vi "Advanced HTML Documentation Wizard.vi"(11 "error in (no error)":errorcluster) -> (15 "error out":errorcluster)   [LabVIEW 2012]
doc: "VI Description text"
uses:
  _Controls and TypeDefs/StartPathLocation_enum.ctl
  _Controls and TypeDefs/InfoFromOldHTML_cluster.ctl
  _Controls and TypeDefs/UserDialogStates.ctl
  <vilib>/Platform/browser.llb/Open URL in Default Browser (string).vi
  <vilib>/Platform/browser.llb/Open URL in Default Browser (path).vi
panel:
  in  "www.labicom.net":bool
  in  "IsChildrenTable?":bool
  in  "Table":string[][](table)=[[" "]] caption="Table with a list of children VIs (that current VI contains)"
  in  "IsScrollableDetails?":bool=TRUE
  in  "Help Button":bool
  out "LV <help> directory?":bool
  in  "IsDetailedHelpLink?":bool=TRUE
  in  "Info extracted from old HTML":T1={"_vi_name_"="", "_vi_description_text_"="", "_vi_controls_and_indicators_descriptions_"="", "_name_of_owning_library_"="", "_owning_library_html_"="", "_Packages_"="Base Package", "_Platforms_"="Windows", "_details_text_"="Put details here", "_example_screenshot_"="", "_example_vi_"="", "_path_to_example_file_"=path "", "IsDetailsON?"=FALSE, "IsOwningLibraryON?"=FALSE, "IsExamplesON?"=FALSE, "IsTableON?"=FALSE, "IsScrollableON?"=FALSE, "IsDetailedHelpLinkON?"=FALSE, "Table Objects array"=[], "Table Descriptions array"=[], "Table Links array"=[], "Start path location"=enum."VI folder"}
  in  "Next_btn":bool caption="Produce VI documentation"
  out "HTML File Path":path
  in  "Cancel Button":bool
  out "Cancelled by User?":bool
  in  "Examples_chkBox":bool
  in  "Details_chkBox":bool=TRUE
  in  "OwningLibrary_chkBox":bool caption="Owning Library/Palette Information"
  in  "Name of Owning Library":string="Put a name here" caption="Name of Owning Library or Palette"
  in  "Path to Owning Library":string caption="Path to Owning Library or Palette"
  in  "Names of Packages":string="Base Package" caption="Names of libraries/packages that this VI requires for its operation"
  in  "Names of Platforms":string="Windows" caption="Names of platforms that this VI supports"
  in  "Details":string="Put details here"
  in  "Image Path for Example":string caption="Path to the image file for Example category"
  in  "Example VI name":string
  in  "Example VI Path":path
  in  "VI Description":string caption="VI Description (with HTML tags)"
  in  "Start path location":T2
  in  "Documentable VI Path":path
  # "Configure VI Documentation Layout"
  # "Additional layout elements for LabVIEW help"
  # "Caution: place <_caution_> into your text"
  # "Note: place <_note_> into your text"
  # "Tip: place <_tip_> into your text"
  # "Windows"
  # "Platform: enclose platform name between\n<_platform_> and </_platform_> tags"
  # "bold"
  # "Text in bold: enclose such text between\n<B> and </B> tags"
  # "Attention!"
  # "Caution Text: enclose such text between \n<_caution_text_> and </_caution_text_> tags"
  # "vigods.com"
  # "Link: place relative path in place of '_path_' and\ntext in place of '_text_' and insert resulting string\nwherever you need: \n<a href=\"_path_\">_text_</a>"
  # "monospace"
  # "Monospace: enclose such text between\n<_monospace_> and </_monospace_> tags"
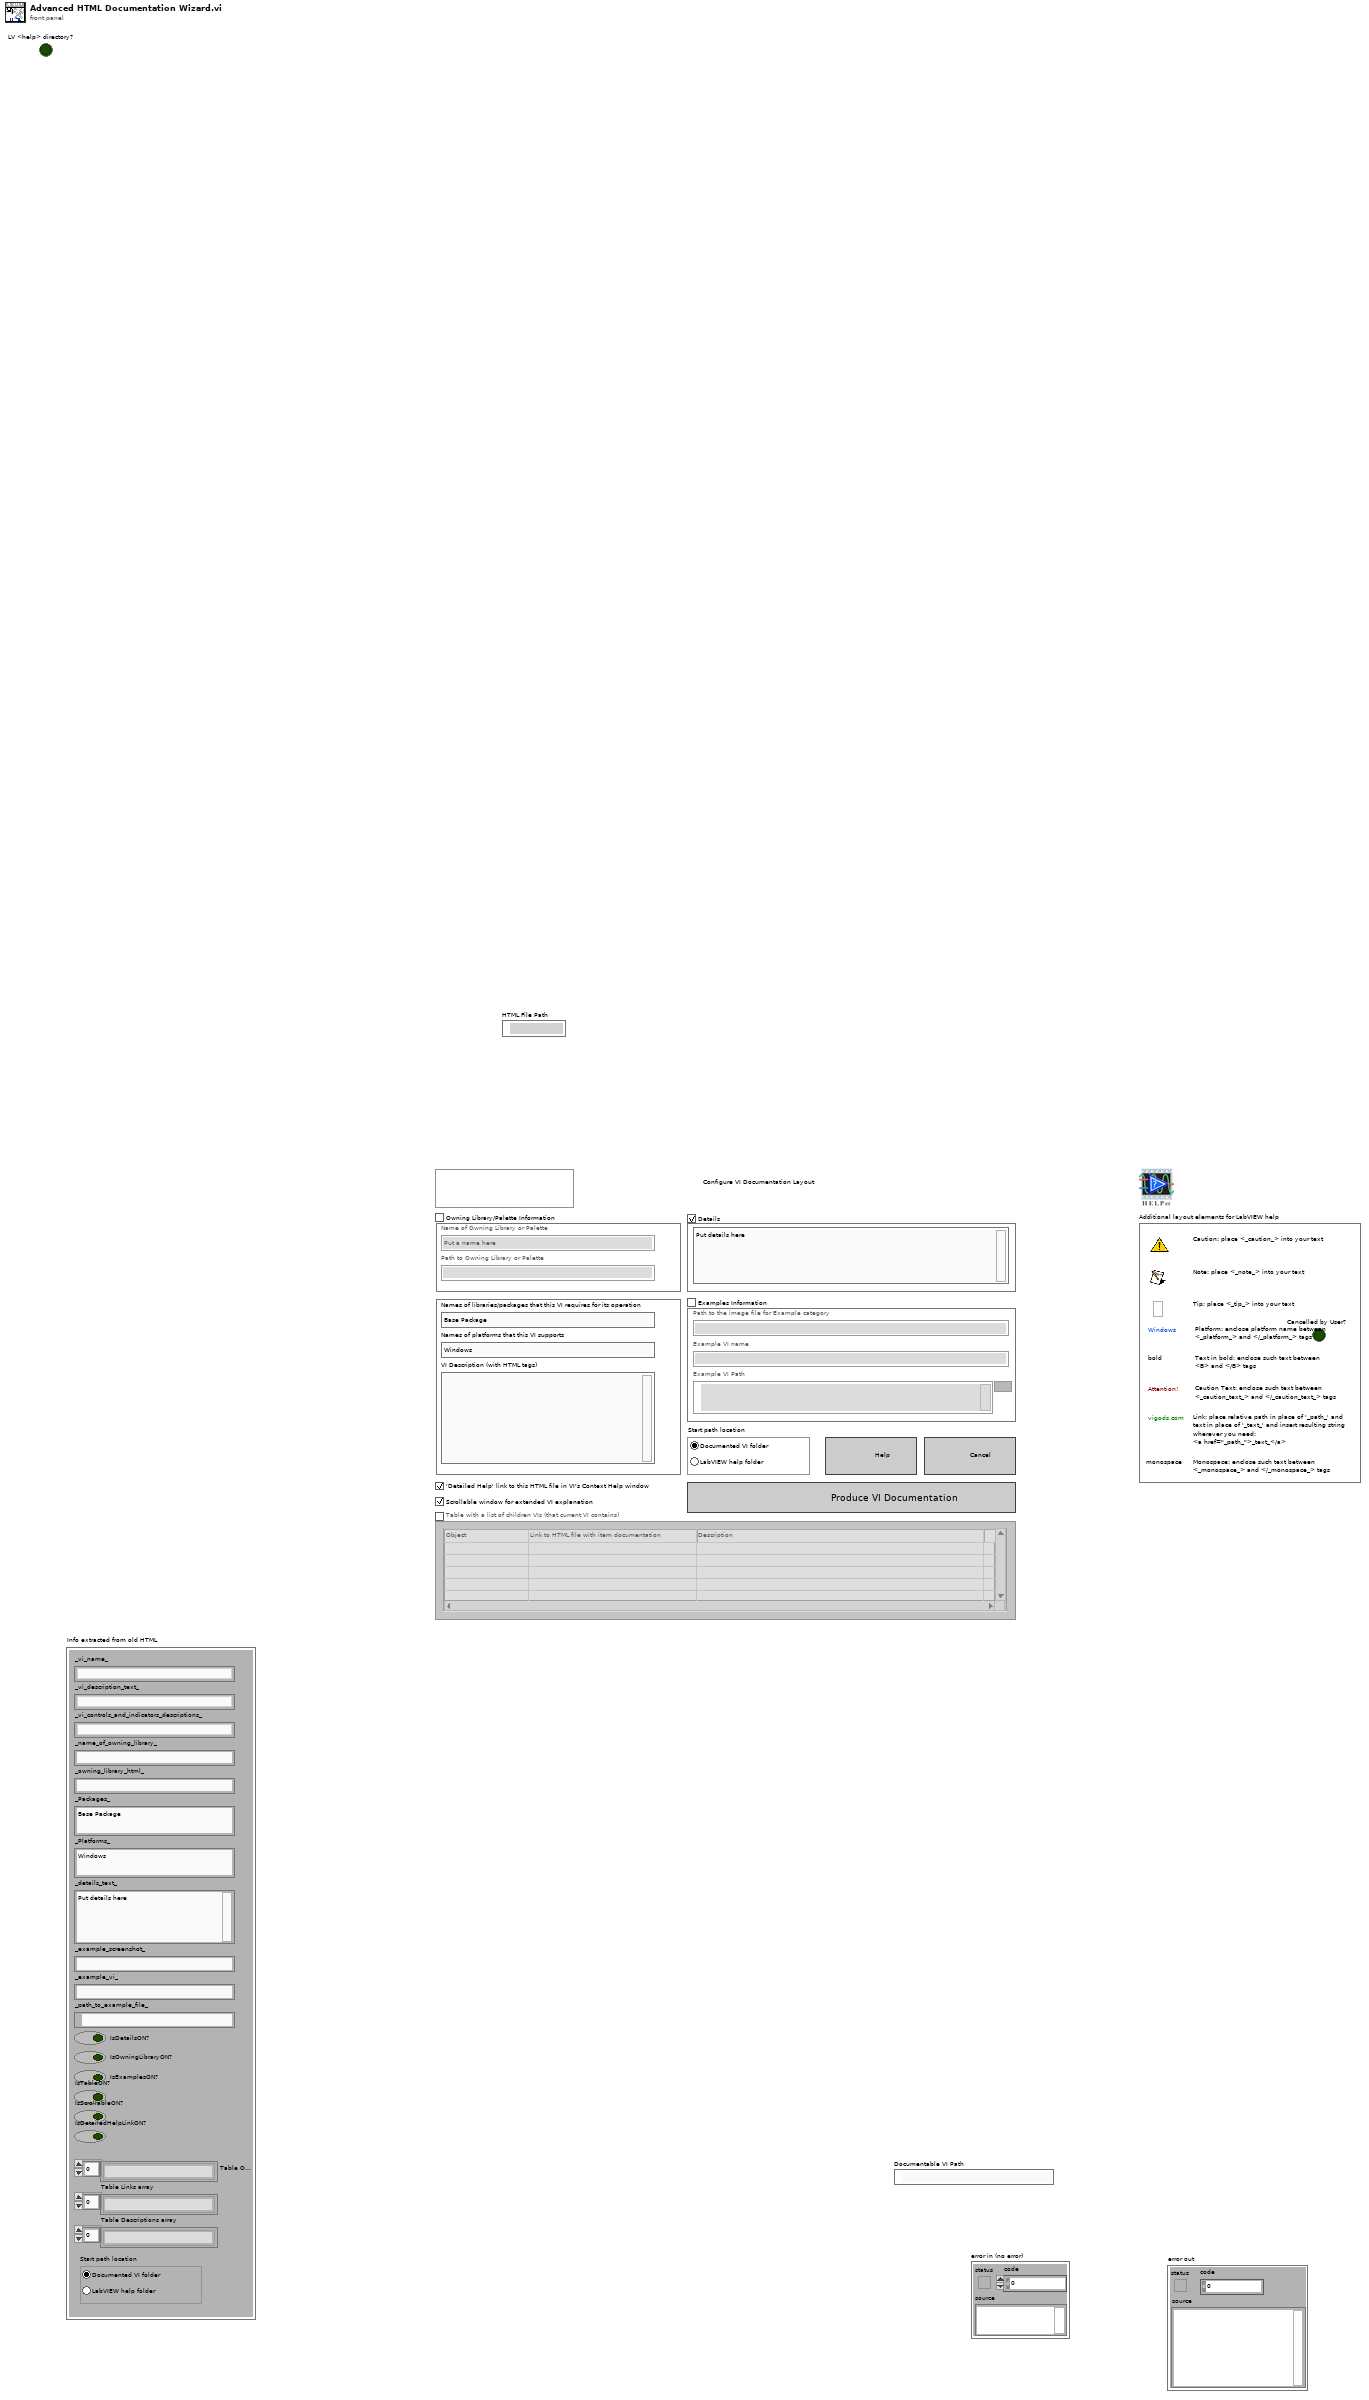
[diagram p1: front panel]
types:
  T1 = typedef "InfoFromOldHTML_cluster.ctl" = cluster{"_vi_name_":string, "_vi_description_text_":string, "_vi_controls_and_indicators_descriptions_":string, "_name_of_owning_library_":string, "_owning_library_html_":string, "_Packages_":string, "_Platforms_":string, "_details_text_":string, "_example_screenshot_":string, "_example_vi_":string, "_path_to_example_file_":path, "IsDetailsON?":bool, "IsOwningLibraryON?":bool, "IsExamplesON?":bool, "IsTableON?":bool, "IsScrollableON?":bool, "IsDetailedHelpLinkON?":bool, "Table Objects array":string[], "Table Descriptions array":string[], "Table Links array":string[], "Start path location":T2}
  T2 = typedef "StartPathLocation_enum.ctl" = enum32{"VI folder", "Help folder"}
  T3 = typedef "UserDialogStates.ctl" = enum16{"Overview", "Known Issues", "Choose parameters", "Update", "Choose HTML file path", "Choose Images directory path", "Decide if there is Context Help", "Choose help hierarchy", "Generate HTML", "Installation", "System Requirements", "Software Support", "Device Support", "Upgrade Issues", "New Features", "Fixed Issues", "Developer", "Contact Support", "Copyright", "Trademarks", "Patents", "Disclaimer", "Save", "Shutdown"}
  T4 = enum8{"Enabled", "Disabled", "Disabled and Grayed Out"}
  T5 = typedef "LVRowAndColumnTypeDef.ctl" = cluster{"Row":i32, "Column":i32}
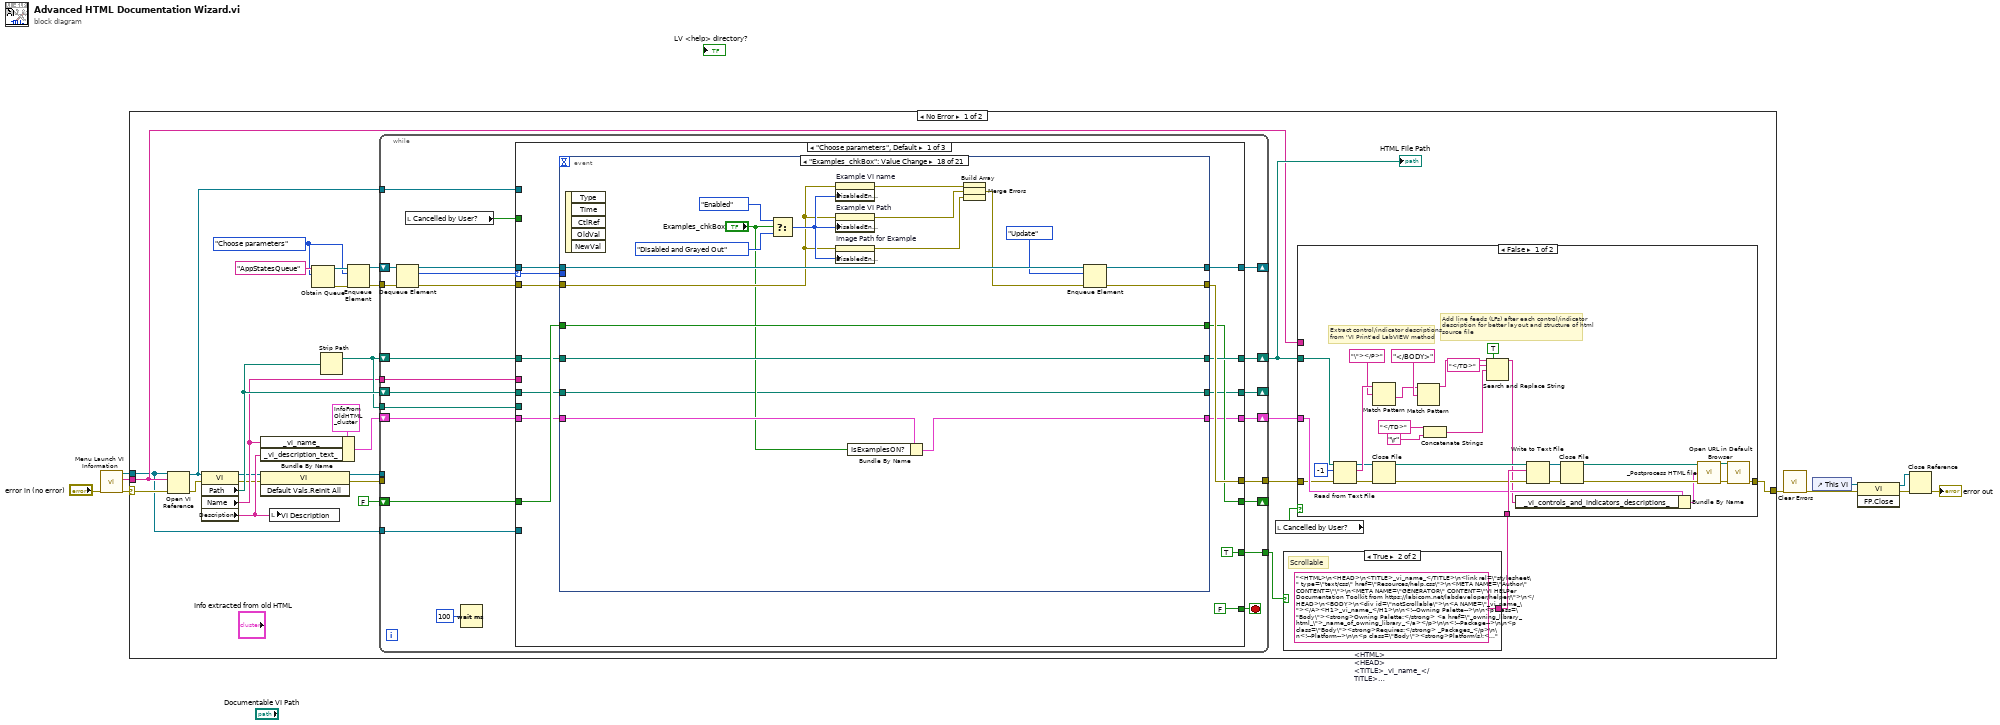
[diagram p0: block diagram]
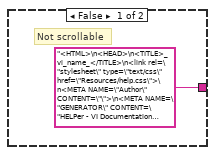
[diagram p2: hidden frame]
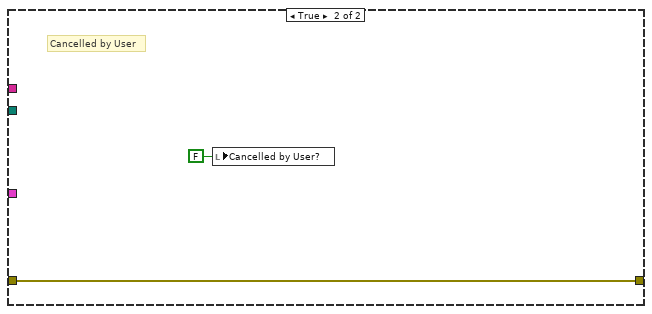
[diagram p3: hidden frame]
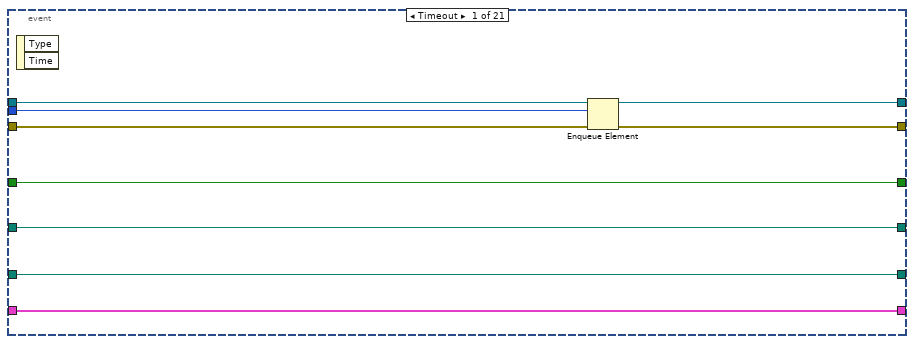
[diagram p4: hidden frame]
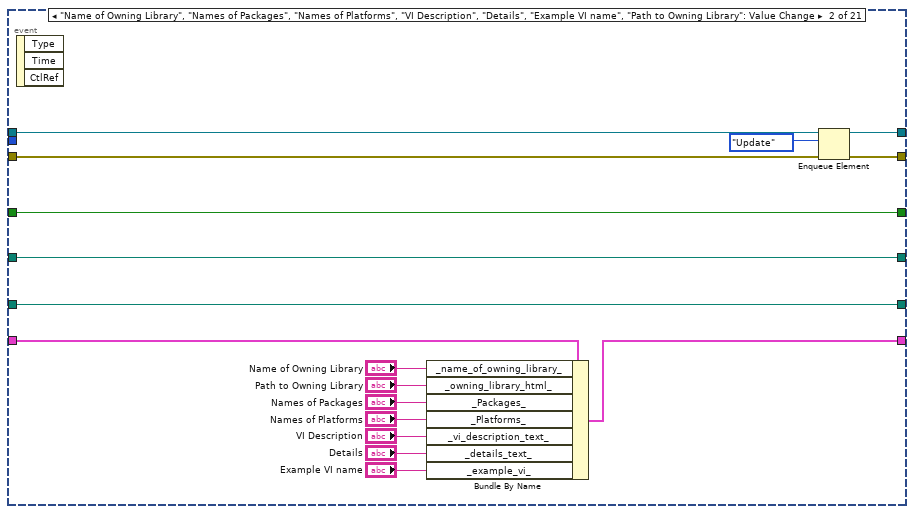
[diagram p5: hidden frame]
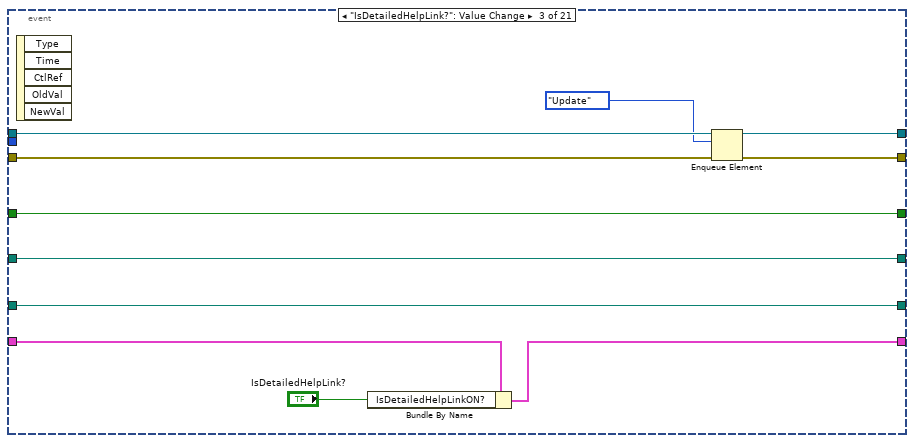
[diagram p6: hidden frame]
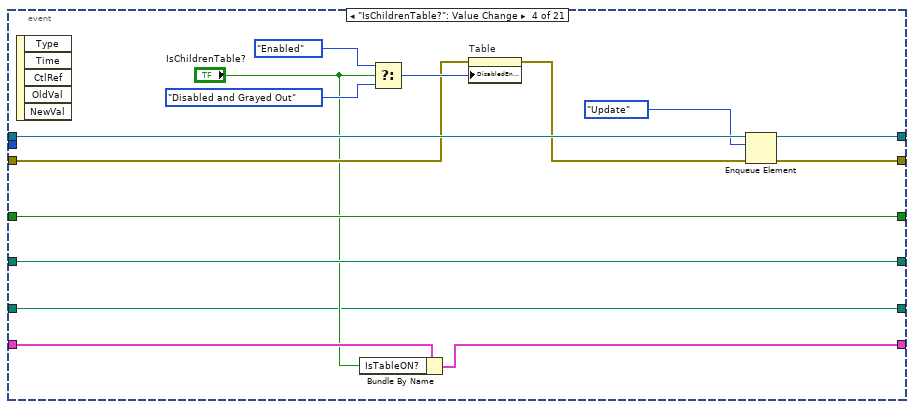
[diagram p7: hidden frame]
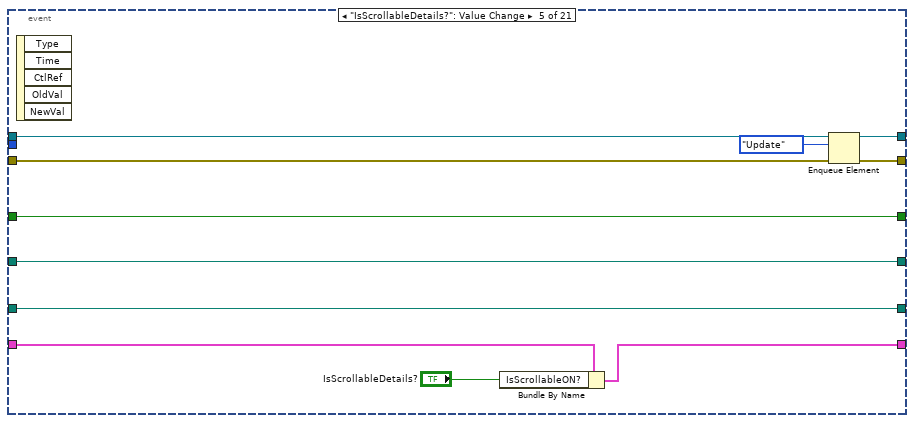
[diagram p8: hidden frame]
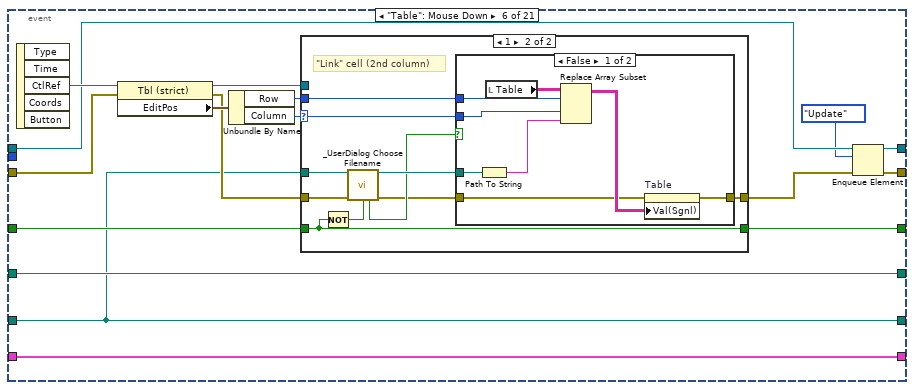
[diagram p9: hidden frame]
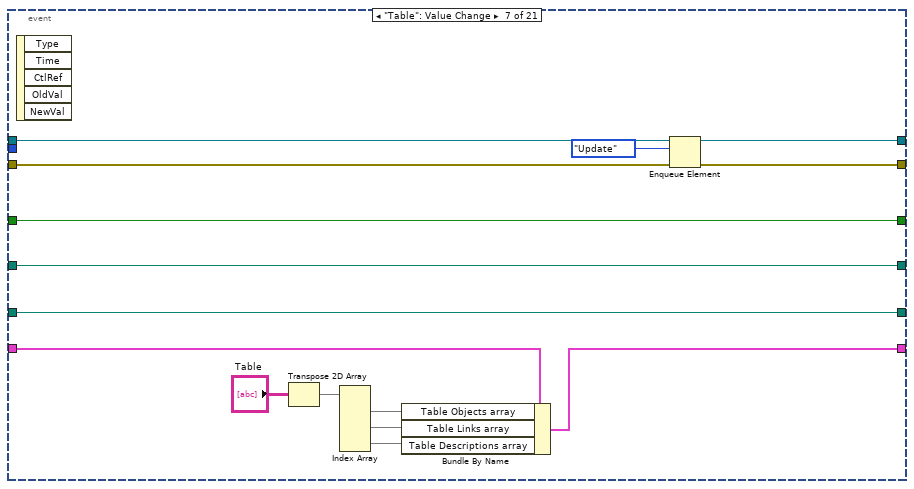
[diagram p12: hidden frame]
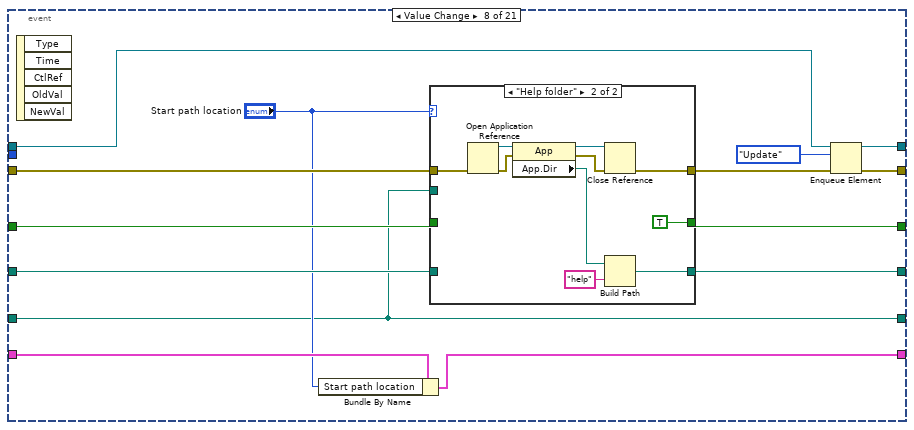
[diagram p13: hidden frame]
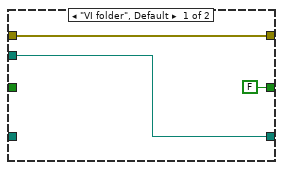
[diagram p14: hidden frame]
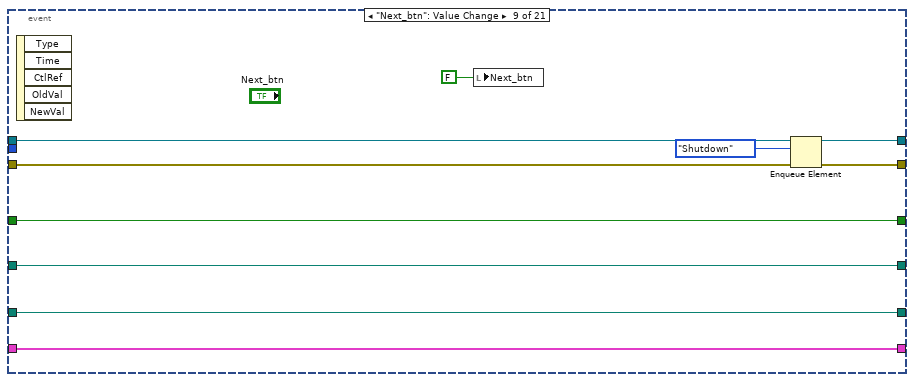
[diagram p15: hidden frame]
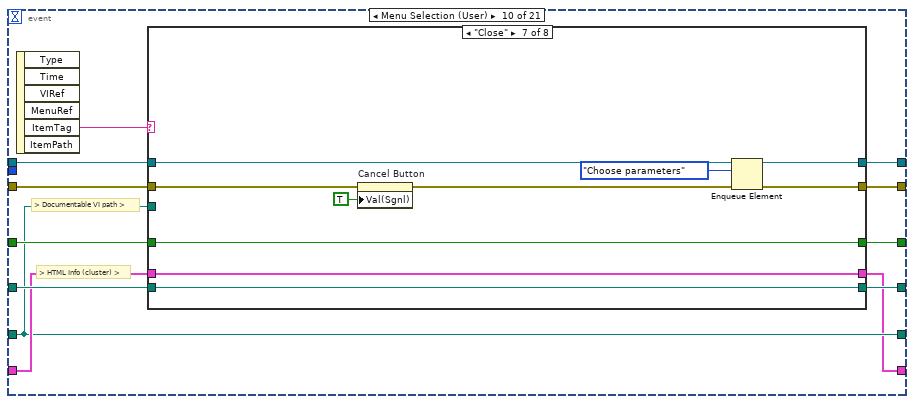
[diagram p16: hidden frame]
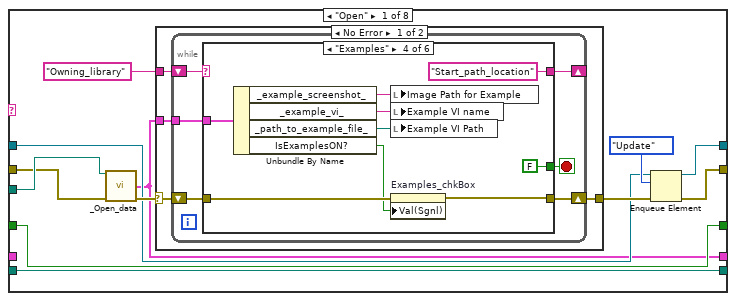
[diagram p17: hidden frame]
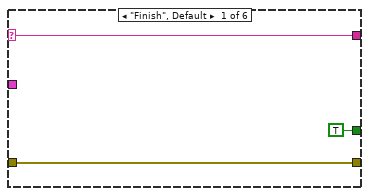
[diagram p18: hidden frame]
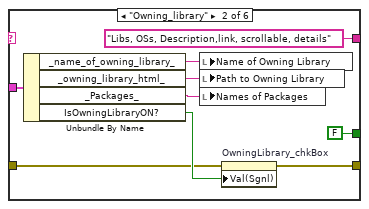
[diagram p19: hidden frame]
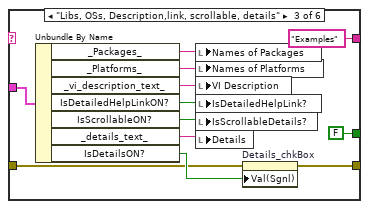
[diagram p20: hidden frame]
diagram:
  n1 = call <vilib>:"Menu Launch VI Information.vi"("error in (no error)"="error in (no error)") -> ("error out"=w7:errorcluster, "Menu Launch:VI"=w9:string, "Menu Launch:App"=w10:refnum<vi>)  [unwired: 8 in]
  n2 = case shown="No Error" w7 {
    selector: w7 -> [w37 w766]
    tunnel: w10 -> [w23 w765]
    tunnel: w9 -> [w24 _]
    tunnel: [w34 w764] -> w2
    frame No Error {
      w13 = UserDialogStates."Choose parameters" ("UserDialogSteps")
      n3 = Open VI Reference(application reference (local)=w23, vi path=w24, error in (no error)=w37) -> (vi reference=w25:refnum<vi>, error out=w39:errorcluster)  [unwired: 3 in]
      n4 = property class="VI"(reference=w25, error in=w39) -> (reference out=w22:refnum<vi>, error out=w20:errorcluster, "Path"=w28:path, "Name"=w26:string, "Description"=w30:string)
      n5 = Bundle By Name(cluster=T1 {"_vi_name_"="", "_vi_description_text_"="", "_vi_controls_and_indicators_descriptions_"="", "_name_of_owning_library_"="", "_owning_library_html_"="", "_Packages_"="Base Package", "_Platforms_"="Windows", "_details_text_"="Put details here", "_example_screenshot_"="", "_example_vi_"="", "_path_to_example_file_"=path "", "IsDetailsON?"=FALSE, "IsOwningLibraryON?"=FALSE, "IsExamplesON?"=FALSE, "IsTableON?"=FALSE, "IsScrollableON?"=FALSE, "IsDetailedHelpLinkON?"=FALSE, "Table Objects array"=[], "Table Descriptions array"=[], "Table Links array"=[], "Start path location"=enum."VI folder"} ("Info extracted from old HTML"), "_vi_name_"=w26, "_vi_description_text_"=w30) -> (w29:T1)
      n6 = invoke class="VI" method="Default Vals.Reinit All"(reference=w22, error in=w20) -> (reference out=w19:refnum<vi>, error out=w21:errorcluster)  [unwired: 1 in, 1 out]
      n7 = local write "VI Description"(w30) -> ()
      n8 = Obtain Queue(name (unnamed)="AppStatesQueue", element data type=w13) -> (queue out=w14:refnum<queue>, error out=w15:errorcluster)  [unwired: 3 in, 1 out]
      n9 = Strip Path(path=w28) -> (stripped path=w27:path)  [unwired: 1 out]
      n10 = Enqueue Element(queue=w14, element=w13, error in (no error)=w15) -> (queue out=w12:refnum<queue>, error out=w11:errorcluster)  [unwired: 1 in, 1 out]
      n11 = while {
        shift-right: [w92] -> _
        shift-left: w12 -> [w75]
        tunnel: w27 -> [w91]
        shift-right: [w90] -> w32
        shift-left: w27 -> [w89]
        shift-right: [w87] -> w35
        shift-left: w29 -> [w88]
        tunnel: w21 -> [_]
        shift-right: [w83] -> _
        shift-left: FALSE -> [w86]
        shift-right: [w82] -> _
        shift-left: w28 -> [w85]
        tunnel: [w84] -> w33
        tunnel: w26 -> [w80]
        tunnel: w25 -> [w79]
        tunnel: w23 -> [w78]
        tunnel: w19 -> [_]
        tunnel: [w77] -> w17
        tunnel: w11 -> [w76]
        stop <- w94 stop-if-true
        n12 = Dequeue Element(queue=w75, error in (no error)=w76) -> (queue out=w72:refnum<queue>, element=w74:T3, error out=w73:errorcluster)  [unwired: 1 in, 1 out]
        n13 = local read "Cancelled by User?"() -> (w81:bool)
        n14 = Wait (ms)(milliseconds to wait=u32 100) -> ()  [unwired: 1 out]
        n15 = case shown="\"Choose parameters\", Default" w74 {
          selector: w74 -> [w108 _ w621]
          tunnel: [FALSE FALSE w633] -> w94
          tunnel: [w107 w611 w627] -> w92
          tunnel: w91 -> [_ _ _]
          tunnel: [w103 w609 w625] -> w90
          tunnel: w89 -> [w104 w609 w628]
          tunnel: w88 -> [w100 w607 w631]
          tunnel: [w95 w607 w630] -> w87
          tunnel: w86 -> [w105 w606 w624]
          tunnel: w85 -> [w97 w608 w632]
          tunnel: [w106 w610 w629] -> w84
          tunnel: [w102 w606 w623] -> w83
          tunnel: [w96 w608 w626] -> w82
          tunnel: w81 -> [_ _ w622]
          tunnel: w80 -> [_ _ w618]
          tunnel: w79 -> [_ _ w620]
          tunnel: w78 -> [_ _ w619]
          tunnel: [TRUE ("IsScrollableDetails?") TRUE ("IsScrollableDetails?") w617] -> w77
          tunnel: w73 -> [w99 w614 w616]
          tunnel: w72 -> [w98 w613 w615]
          frame "Choose parameters", Default {
            n16 = event shown="[17] \"Examples_chkBox\": Value Change" {
              selector: _ -> [_ _ _ _ _ _ _ _ _ _ _ _ _ _ _ _ _ _ _ _ _]
              dyn-events: _ -> [_ _ _ _ _ _ _ _ _ _ _ _ _ _ _ _ _ _ _ _ _]
              timeout: _ -> [_ _ _ _ _ _ _ _ _ _ _ _ _ _ _ _ _ _ _ _ _]
              tunnel: w108 -> [w116 _ _ _ _ _ _ _ _ _ _ _ _ _ _ _ _ _ _ _ _]
              tunnel: [w114 w129 w141 w152 w165 w176 w220 w231 w256 w265 w434 w459 w476 w486 w513 w524 w541 w557 w573 w584 w596] -> w107
              tunnel: w105 -> [w117 w134 w145 w158 w170 w183 w224 w236 w260 w273 w438 w462 w474 w491 w509 w529 w546 w564 w580 w590 w601]
              tunnel: w99 -> [w113 w132 w143 w153 w167 w180 w222 w237 w259 w267 w442 w456 w477 w493 w512 w528 w544 w559 w578 w591 w598]
              tunnel: [w112 w130 w140 w151 w164 w175 w219 w230 w257 w269 w433 w458 w475 w485 w511 w523 w540 w556 w572 w583 w595] -> w106
              tunnel: w104 -> [w118 w135 w146 w157 w169 w181 w225 w239 w261 w271 w441 w465 w473 w492 w510 w532 w547 w565 w579 w589 w602]
              tunnel: [w118 w135 w146 w157 w169 w181 w225 w238 w261 w270 w441 w465 w473 w492 w510 w532 w547 w565 w579 w589 w602] -> w103
              tunnel: [w117 w134 w145 w158 w170 w182 w224 w235 w260 w272 w438 w462 w474 w491 w509 w529 w546 w564 w580 w590 w601] -> w102
              tunnel: w100 -> [w110 w128 w139 w150 w172 w173 w212 w229 w253 w268 w431 w453 w482 w483 w517 w522 w539 w555 w570 w581 w592]
              tunnel: w98 -> [w115 w133 w144 w156 w166 w178 w223 w233 w258 w266 w437 w460 w478 w490 w514 w527 w545 w561 w575 w586 w597]
              tunnel: w97 -> [w111 w127 w137 w148 w163 w174 w213 w227 w254 w264 w432 w454 w472 w484 w508 w520 w537 w553 w571 w582 w593]
              tunnel: [w111 w127 w137 w148 w163 w174 w213 w227 w254 w264 w432 w454 w472 w484 w508 w520 w537 w553 w571 w582 w593] -> w96
              tunnel: [w110 w126 w136 w147 w162 w173 w211 w226 w253 w263 w431 w453 w480 w483 w507 w519 w536 w552 w570 w581 w592] -> w95
              event Timeout {
                n17 = event-data() -> ()  [unwired: 1 in, 2 out]
                n18 = Enqueue Element(queue=w115, element=w116, error in (no error)=w113) -> (queue out=w114:refnum<queue>, error out=w112:errorcluster)  [unwired: 1 in, 1 out]
              }
              event "Name of Owning Library", "Names of Packages", "Names of Platforms", "VI Description", "Details", "Example VI name", "Path to Owning Library": Value Change {
                n19 = event-data() -> ()  [unwired: 1 in, 3 out]
                n20 = Bundle By Name(cluster=w128, "_name_of_owning_library_"="Name of Owning Library", "_owning_library_html_"="Path to Owning Library", "_Packages_"="Names of Packages", "_Platforms_"="Names of Platforms", "_vi_description_text_"="VI Description", "_details_text_"="Details", "_example_vi_"="Example VI name") -> (w126:T1)
                n21 = Enqueue Element(queue=w133, element=UserDialogStates."Update" ("UserDialogSteps"), error in (no error)=w132) -> (queue out=w129:refnum<queue>, error out=w130:errorcluster)  [unwired: 1 in, 1 out]
              }
              event "IsDetailedHelpLink?": Value Change {
                n22 = event-data() -> ()  [unwired: 1 in, 5 out]
                n23 = Bundle By Name(cluster=w139, "IsDetailedHelpLinkON?"="IsDetailedHelpLink?") -> (w136:T1)
                n24 = Enqueue Element(queue=w144, element=UserDialogStates."Update" ("UserDialogSteps"), error in (no error)=w143) -> (queue out=w141:refnum<queue>, error out=w140:errorcluster)  [unwired: 1 in, 1 out]
              }
              event "IsChildrenTable?": Value Change {
                n25 = event-data() -> ()  [unwired: 1 in, 5 out]
                n26 = Bundle By Name(cluster=w150, "IsTableON?"="IsChildrenTable?") -> (w147:T1)
                n27 = Select(t=T4."Enabled" ("Disabled"), s="IsChildrenTable?", f=T4."Disabled and Grayed Out") -> (s? t:f=w159:T4)
                n28 = property on="Table" class="Tbl (strict)"(error in=w153, "DisabledEnum"=w159) -> (error out=w154:errorcluster)  [unwired: 1 in, 1 out]
                n29 = Enqueue Element(queue=w156, element=UserDialogStates."Update" ("UserDialogSteps"), error in (no error)=w154) -> (queue out=w152:refnum<queue>, error out=w151:errorcluster)  [unwired: 1 in, 1 out]
              }
              event "IsScrollableDetails?": Value Change {
                n30 = event-data() -> ()  [unwired: 1 in, 5 out]
                n31 = Bundle By Name(cluster=w172, "IsScrollableON?"="IsScrollableDetails?") -> (w162:T1)
                n32 = Enqueue Element(queue=w166, element=UserDialogStates."Update" ("UserDialogSteps"), error in (no error)=w167) -> (queue out=w165:refnum<queue>, error out=w164:errorcluster)  [unwired: 1 in, 1 out]
              }
              event "Table": Mouse Down {
                n33 = event-data() -> ("CtlRef"=w184:refnum<vi>)  [unwired: 1 in, 4 out]
                n34 = property class="Tbl (strict)"(reference=w184, error in=w180) -> (reference out=w187:refnum<vi>, error out=w186:errorcluster, "EditPos"=w189:T5)
                n35 = Unbundle By Name(w189) -> ("Row"=w185:i32, "Column"=w188:i32)
                n36 = case shown="1" w188 {
                  selector: w188 -> [_ w197]
                  tunnel: w183 -> [w190 w196]
                  tunnel: w174 -> [_ w201]
                  tunnel: w187 -> [_ _]
                  tunnel: w186 -> [w191 w199]
                  tunnel: w185 -> [_ w198]
                  tunnel: [w191 w192] -> w179
                  tunnel: [w190 w196] -> w182
                  frame 0, Default {
                  }
                  frame 1 {
                    # "\"Link\" cell (2nd column)"
                    n37 = Not(x=w196) -> (.not. x?=w195:bool)
                    n38 = call "_UserDialog Choose Filename.vi"("VI Default Path"=w201, "error in (no error)"=w199, "Not In <help> directory? (Yes: T)"=w195) -> ("HTML File Path"=w200:path, "Cancelled by User?"=w194:bool, "error out"=w193:errorcluster)  [unwired: 8 in, 2 out]
                    n39 = case shown="False" w194 {
                      tunnel: w200 -> [w209 _]
                      tunnel: w198 -> [w207 _]
                      tunnel: w197 -> [w206 _]
                      tunnel: w193 -> [w203 w210]
                      tunnel: [w202 w210] -> w192
                      frame False {
                        n40 = Path To String(path=w209) -> (string=w205:string)
                        n41 = local read "Table"() -> (w208:string[][])
                        n42 = Replace Array Subset(array=w208, new element=w205, index (row)=w207, index (col)=w206) -> (w204:string[][])
                        n43 = property on="Table" class="Tbl (strict)"(error in=w203, "Val(Sgnl)"=w204) -> (error out=w202:errorcluster)  [unwired: 1 in, 1 out]
                      }
                      frame True {
                      }
                    }
                  }
                }
                n44 = Enqueue Element(queue=w178, element=UserDialogStates."Update", error in (no error)=w179) -> (queue out=w176:refnum<queue>, error out=w175:errorcluster)  [unwired: 1 in, 1 out]
              }
              event "Table": Value Change {
                n45 = event-data() -> ()  [unwired: 1 in, 5 out]
                n46 = Transpose 2D Array(2D array="Table") -> (transposed array=w216:string[][])
                n47 = Index Array(array=w216) -> (element #1=w215:string[], element #2=w218:string[], element #3=w214:string[])  [unwired: 6 in]
                n48 = Bundle By Name(cluster=w212, "Table Objects array"=w215, "Table Links array"=w218, "Table Descriptions array"=w214) -> (w211:T1)
                n49 = Enqueue Element(queue=w223, element=UserDialogStates."Update" ("UserDialogSteps"), error in (no error)=w222) -> (queue out=w220:refnum<queue>, error out=w219:errorcluster)  [unwired: 1 in, 1 out]
              }
              event Value Change {
                n50 = event-data() -> ()  [unwired: 1 in, 5 out]
                n51 = Bundle By Name(cluster=w229, "Start path location"="Start path location") -> (w226:T1)
                n52 = case shown="\"Help folder\"" "Start path location" {
                  tunnel: w239 -> [_ _]
                  tunnel: [w242 w246] -> w238
                  tunnel: w237 -> [w241 w245]
                  tunnel: [w241 w244] -> w234
                  tunnel: w227 -> [w242 _]
                  tunnel: w236 -> [_ _]
                  tunnel: [FALSE TRUE] -> w235
                  frame "VI folder", Default {
                  }
                  frame "Help folder" {
                    n53 = Open Application Reference(8:w245) -> (0:w248:errorcluster, 3:w247:refnum<vi>)  [unwired: 3 in]
                    n54 = property class="App"(reference=w247, error in=w248) -> (reference out=w249:refnum<vi>, error out=w250:errorcluster, "App.Dir"=w251:path)
                    n55 = Close Reference(reference=w249, error in (no error)=w250) -> (error out=w244:errorcluster)
                    n56 = Build Path(base path=w251, name or relative path="help") -> (appended path=w246:path)
                  }
                }
                n57 = Enqueue Element(queue=w233, element=UserDialogStates."Update" ("UserDialogSteps"), error in (no error)=w234) -> (queue out=w231:refnum<queue>, error out=w230:errorcluster)  [unwired: 1 in, 1 out]
              }
              event "Next_btn": Value Change {
                n58 = event-data() -> ()  [unwired: 1 in, 5 out]
                n59 = local write "Next_btn"(FALSE ("Next Button")) -> ()
                n60 = Enqueue Element(queue=w258, element=UserDialogStates."Shutdown" ("UserDialogSteps"), error in (no error)=w259) -> (queue out=w256:refnum<queue>, error out=w257:errorcluster)  [unwired: 1 in, 1 out]
              }
              event Menu Selection (User) {
                # "> HTML Info (cluster) >"
                # "> Documentable VI path >"
                n61 = event-data() -> ("ItemTag"=w274:string)  [unwired: 1 in, 5 out]
                n62 = case shown="\"Close\"" w274 {
                  tunnel: w273 -> [w284 w363 w376 w390 w400 w410 w422 w430]
                  tunnel: [w284 w363 w376 w390 w400 w410 w422 w430] -> w272
                  tunnel: w271 -> [w286 w362 w375 w389 w399 w409 w421 w429]
                  tunnel: [w286 w362 w375 w389 w399 w409 w421 w429] -> w270
                  tunnel: w267 -> [w278 w357 w374 w391 w401 w411 w419 w427]
                  tunnel: [w281 w354 w368 w387 w397 w407 w415 w425] -> w269
                  tunnel: [w280 w351 w367 w385 w394 w406 w416 w426] -> w265
                  tunnel: w268 -> [_ w350 w364 w383 w393 w403 w413 w423]
                  tunnel: w264 -> [w282 w361 w373 _ _ _ _ _]
                  tunnel: w266 -> [w276 w353 w365 w384 w396 w404 w418 w428]
                  tunnel: [w275 w350 w364 w383 w393 w403 w413 w423] -> w263
                  frame "Open" {
                    n63 = call "_Open_data.vi"("Documented VI path"=w282, "error in"=w278) -> ("XML Info cluster"=w275:T1, "error out"=w283:errorcluster)  [unwired: 12 in]
                    n64 = case shown="No Error" w283 {
                      selector: w283 -> [w287 w348]
                      tunnel: w275 -> [w290 _]
                      tunnel: "Owning_library" -> [w289 _]
                      tunnel: [w288 w347] -> w277
                      frame No Error {
                        n65 = while {
                          tunnel: w290 -> [w295]
                          shift-right: [w291] -> _
                          shift-left: w289 -> [w296]
                          shift-right: [w292] -> w288
                          shift-left: w287 -> [w293]
                          stop <- w294 stop-if-true
                          n66 = case shown="\"Examples\"" w296 {
                            selector: w296 -> [w298 _ _ _ _ _]
                            tunnel: w295 -> [_ w308 w309 w328 w334 w344]
                            tunnel: [TRUE FALSE FALSE FALSE FALSE FALSE] -> w294
                            tunnel: w293 -> [w297 w302 w312 w324 w332 w337]
                            tunnel: [w297 w301 w311 w323 w331 w336] -> w292
                            tunnel: [w298 "Libs, OSs, Description,link, scrollable, details" "Examples" "Start_path_location" "Table" "Finish"] -> w291
                            frame "Finish", Default {
                            }
                            frame "Owning_library" {
                              n67 = Unbundle By Name(w308) -> ("_name_of_owning_library_"=w307:string, "_owning_library_html_"=w306:string, "_Packages_"=w305:string, "IsOwningLibraryON?"=w304:bool)
                              n68 = local write "Name of Owning Library"(w307) -> ()
                              n69 = local write "Path to Owning Library"(w306) -> ()
                              n70 = local write "Names of Packages"(w305) -> ()
                              n71 = property on="OwningLibrary_chkBox" class="Bool (strict)"(error in=w302, "Val(Sgnl)"=w304) -> (error out=w301:errorcluster)  [unwired: 1 in, 1 out]
                            }
                            frame "Libs, OSs, Description,link, scrollable, details" {
                              n72 = Unbundle By Name(w309) -> ("_Packages_"=w318:string, "_Platforms_"=w317:string, "_vi_description_text_"=w316:string, "IsDetailedHelpLinkON?"=w320:bool, "IsScrollableON?"=w319:bool, "_details_text_"=w314:string, "IsDetailsON?"=w313:bool)
                              n73 = local write "Names of Packages"(w318) -> ()
                              n74 = local write "Names of Platforms"(w317) -> ()
                              n75 = local write "VI Description"(w316) -> ()
                              n76 = local write "IsDetailedHelpLink?"(w320) -> ()
                              n77 = local write "IsScrollableDetails?"(w319) -> ()
                              n78 = local write "Details"(w314) -> ()
                              n79 = property on="Details_chkBox" class="Bool (strict)"(error in=w312, "Val(Sgnl)"=w313) -> (error out=w311:errorcluster)  [unwired: 1 in, 1 out]
                            }
                            frame "Examples" {
                              n80 = Unbundle By Name(w328) -> ("_example_screenshot_"=w326:string, "_example_vi_"=w327:string, "_path_to_example_file_"=w325:path, "IsExamplesON?"=w322:bool)
                              n81 = local write "Image Path for Example"(w326) -> ()
                              n82 = local write "Example VI name"(w327) -> ()
                              n83 = local write "Example VI Path"(w325) -> ()
                              n84 = property on="Examples_chkBox" class="Bool (strict)"(error in=w324, "Val(Sgnl)"=w322) -> (error out=w323:errorcluster)  [unwired: 1 in, 1 out]
                            }
                            frame "Start_path_location" {
                              n85 = Unbundle By Name(w334) -> ("Start path location"=w333:T2)
                              n86 = property on="Start path location" class="RadioBtnsControl (strict)"(error in=w332, "Val(Sgnl)"=w333) -> (error out=w331:errorcluster)  [unwired: 1 in, 1 out]
                            }
                            frame "Table" {
                              n87 = Unbundle By Name(w344) -> ("Table Objects array"=w343:string[], "Table Links array"=w342:string[], "Table Descriptions array"=w341:string[], "IsTableON?"=w338:bool)
                              n88 = Build Array(w343, w342, w341) -> (w340:string[][])
                              n89 = property on="IsChildrenTable?" class="Bool (strict)"(error in=w337, "Val(Sgnl)"=w338) -> (error out=w336:errorcluster)  [unwired: 1 in, 1 out]
                              n90 = Transpose 2D Array(2D array=w340) -> (transposed array=w339:string[][])
                              n91 = local write "Table"(w339) -> ()
                            }
                          }
                        }
                      }
                      frame Error {
                        n92 = One Button Dialog(message="Error! There is no any HELPer file associated with\ndocumented VI.") -> ()  [unwired: 1 in, 1 out]
                        n93 = call <vilib>:"Clear Errors.vi"("error in (no error)"=w348) -> ("error out"=w347:errorcluster)  [unwired: 6 in]
                      }
                    }
                    n94 = Enqueue Element(queue=w276, element=UserDialogStates."Update" ("UserDialogSteps"), error in (no error)=w277) -> (queue out=w280:refnum<queue>, error out=w281:errorcluster)  [unwired: 1 in, 1 out]
                  }
                  frame "Save_to_VI_directory" {
                    n95 = Path To String(path=w361) -> (string=w360:string)
                    n96 = Concatenate Strings(w360, ".vihlp" ("string")) -> (w358:string)
                    n97 = String To Path(string=w358) -> (path=w356:path)
                    n98 = call "_Save_data.vi"("vihlp Path"=w356, "Info extracted from old HTML"=w350, "error in"=w357) -> ("error out"=w355:errorcluster)  [unwired: 12 in]
                    n99 = Enqueue Element(queue=w353, element=UserDialogStates."Update" ("UserDialogSteps"), error in (no error)=w355) -> (queue out=w351:refnum<queue>, error out=w354:errorcluster)  [unwired: 1 in, 1 out]
                  }
                  frame "Save_to_project_directory" {
                    n100 = call "_Build VIHLP path.vi"("Documented VI path"=w373, "error in"=w374) -> ("Path to VIHLP file"=w371:path, "error out"=w372:errorcluster)  [unwired: 12 in]
                    n101 = Path To String(path=w371) -> (string=w370:string)
                    n102 = case shown="\"Any legal path\", Default" w370 {
                      tunnel: [w378 w382] -> w369
                      tunnel: w364 -> [_ w379]
                      tunnel: w372 -> [w378 w381]
                      tunnel: w371 -> [_ w380]
                      frame "<Not A Path>.vihlp" {
                        n103 = One Button Dialog(message="Documentation file for this VI wasn't saved.\nDocumented VI is not under any \nLabVIEW project hierarchy.\nPlace it inside LabVIEW project or \nsave with 'Save to VI Directory' option.") -> ()  [unwired: 1 in, 1 out]
                      }
                      frame "Any legal path", Default {
                        n104 = call "_Save_data.vi"("vihlp Path"=w380, "Info extracted from old HTML"=w379, "error in"=w381) -> ("error out"=w382:errorcluster)  [unwired: 12 in]
                      }
                    }
                    n105 = Enqueue Element(queue=w365, element=UserDialogStates."Update" ("UserDialogSteps"), error in (no error)=w369) -> (queue out=w367:refnum<queue>, error out=w368:errorcluster)  [unwired: 1 in, 1 out]
                  }
                  frame "HELPer_help" {
                    n106 = call "Read me and Help.vi"("path"=path "viGods.com/HELPer/helper.html", "error in"=w391) -> ("error out"=w388:errorcluster)  [unwired: 13 in]
                    n107 = Enqueue Element(queue=w384, element=UserDialogStates."Update" ("UserDialogSteps"), error in (no error)=w388) -> (queue out=w385:refnum<queue>, error out=w387:errorcluster)  [unwired: 1 in, 1 out]
                  }
                  frame "Help_for_Wizard" {
                    n108 = call "Read me and Help.vi"("path"=path "viGods.com/HELPer/advanced.html", "error in"=w401) -> ("error out"=w398:errorcluster)  [unwired: 13 in]
                    n109 = Enqueue Element(queue=w396, element=UserDialogStates."Update" ("UserDialogSteps"), error in (no error)=w398) -> (queue out=w394:refnum<queue>, error out=w397:errorcluster)  [unwired: 1 in, 1 out]
                  }
                  frame "About_HELPer" {
                    n110 = call "Read me and Help.vi"("path"=path "viGods.com/HELPer/about.html", "error in"=w411) -> ("error out"=w408:errorcluster)  [unwired: 13 in]
                    n111 = Enqueue Element(queue=w404, element=UserDialogStates."Update" ("UserDialogSteps"), error in (no error)=w408) -> (queue out=w406:refnum<queue>, error out=w407:errorcluster)  [unwired: 1 in, 1 out]
                  }
                  frame "Close" {
                    n112 = property on="Cancel Button" class="Bool (strict)"(error in=w419, "Val(Sgnl)"=TRUE ("Value (Signaling)")) -> (error out=w417:errorcluster)  [unwired: 1 in, 1 out]
                    n113 = Enqueue Element(queue=w418, element=UserDialogStates."Choose parameters" ("UserDialogSteps"), error in (no error)=w417) -> (queue out=w416:refnum<queue>, error out=w415:errorcluster)  [unwired: 1 in, 1 out]
                  }
                  frame "False", Default {
                    n114 = Enqueue Element(queue=w428, element=UserDialogStates."Update" ("UserDialogSteps"), error in (no error)=w427) -> (queue out=w426:refnum<queue>, error out=w425:errorcluster)  [unwired: 1 in, 1 out]
                  }
                }
              }
              event "Path to Owning Library": Mouse Down {
                n115 = event-data() -> ()  [unwired: 1 in, 2 out]
                n116 = local read "Name of Owning Library"() -> (w447:string)
                n117 = Concatenate Strings(w447, ".html" ("string")) -> (w446:string)
                n118 = Not(x=w438) -> (.not. x?=w439:bool)
                n119 = call "_UserDialog Choose Filename.vi"("VI Default Path"=w441, "Default file name"=w446, "error in (no error)"=w442, "Not In <help> directory? (Yes: T)"=w439) -> ("HTML File Path"=w444:path, "Cancelled by User?"=w440:bool, "error out"=w443:errorcluster)  [unwired: 7 in, 2 out]
                n120 = case shown="False" w440 {
                  tunnel: w444 -> [w451 _]
                  tunnel: w443 -> [w449 w452]
                  tunnel: [w448 w452] -> w436
                  tunnel: w441 -> [_ _]
                  frame False {
                    n121 = Path To String(path=w451) -> (string=w450:string)
                    n122 = property on="Path to Owning Library" class="Str"(error in=w449, "Val(Sgnl)"=w450) -> (error out=w448:errorcluster)  [unwired: 1 in, 1 out]
                  }
                  frame True {
                  }
                }
                n123 = Enqueue Element(queue=w437, element=UserDialogStates."Update" ("UserDialogSteps"), error in (no error)=w436) -> (queue out=w434:refnum<queue>, error out=w433:errorcluster)  [unwired: 1 in, 1 out]
              }
              event "Image Path for Example": Mouse Down {
                n124 = event-data() -> ()  [unwired: 1 in, 2 out]
                n125 = Not(x=w462) -> (.not. x?=w463:bool)
                n126 = call "_UserDialog Choose Filename.vi"("VI Default Path"=w465, "Default file name"="ExampleImage.png", "Not In <help> directory? (Yes: T)"=w463) -> ("HTML File Path"=w461:path, "Cancelled by User?"=w464:bool)  [unwired: 8 in, 3 out]
                n127 = case shown="False" w464 {
                  tunnel: w461 -> [w470 _]
                  tunnel: w456 -> [w468 w471]
                  tunnel: [w467 w471] -> w455
                  frame False {
                    n128 = Path To String(path=w470) -> (string=w469:string)
                    n129 = property on="Image Path for Example" class="Str"(error in=w468, "Val(Sgnl)"=w469) -> (error out=w467:errorcluster)  [unwired: 1 in, 1 out]
                  }
                  frame True {
                  }
                }
                n130 = Enqueue Element(queue=w460, element=UserDialogStates."Update" ("UserDialogSteps"), error in (no error)=w455) -> (queue out=w459:refnum<queue>, error out=w458:errorcluster)  [unwired: 1 in, 1 out]
              }
              event "Image Path for Example": Value Change {
                n131 = event-data() -> ()  [unwired: 1 in, 5 out]
                n132 = Bundle By Name(cluster=w482, "_example_screenshot_"="Image Path for Example") -> (w480:T1)
                n133 = Enqueue Element(queue=w478, element=UserDialogStates."Update" ("UserDialogSteps"), error in (no error)=w477) -> (queue out=w476:refnum<queue>, error out=w475:errorcluster)  [unwired: 1 in, 1 out]
              }
              event "Example VI Path": Mouse Down {
                n134 = event-data() -> ()  [unwired: 1 in, 4 out]
                n135 = disable-structure shown="Enabled" {
                  disable-tunnel: [w504 w506] -> w494
                  disable-tunnel: w491 -> [w496 _]
                  disable-tunnel: w493 -> [w495 w506]
                  disable-tunnel: w490 -> [_ w505]
                  disable-tunnel: [_ w505] -> w489
                  frame Disabled {
                    n136 = Open Application Reference(8:w495) -> (0:w501:errorcluster, 3:w502:refnum<vi>)  [unwired: 3 in]
                    n137 = property class="App"(reference=w502, error in=w501) -> (reference out=w500:refnum<vi>, error out=w499:errorcluster, "App.Dir"=w498:path)
                    n138 = Close Reference(reference=w500, error in (no error)=w499) -> (error out=w504:errorcluster)
                    n139 = Build Path(base path=w498, name or relative path="help") -> (appended path=w503:path)
                    n140 = Select(s=w496, f=w503) -> ()  [unwired: 1 in, 1 out]
                  }
                  frame Enabled {
                  }
                }
                n141 = property on="Example VI Path" class="Path"(error in=w494, "StartPath"=w492) -> (error out=w488:errorcluster)  [unwired: 1 in, 1 out]
                n142 = Enqueue Element(queue=w489, element=UserDialogStates."Update" ("UserDialogSteps"), error in (no error)=w488) -> (queue out=w486:refnum<queue>, error out=w485:errorcluster)  [unwired: 1 in, 1 out]
              }
              event "Example VI Path": Value Change {
                n143 = event-data() -> ()  [unwired: 1 in, 5 out]
                n144 = Bundle By Name(cluster=w517, "_path_to_example_file_"="Example VI Path") -> (w507:T1)
                n145 = Enqueue Element(queue=w514, element=UserDialogStates."Update" ("UserDialogSteps"), error in (no error)=w512) -> (queue out=w513:refnum<queue>, error out=w511:errorcluster)  [unwired: 1 in, 1 out]
              }
              event "OwningLibrary_chkBox": Value Change {
                n146 = event-data() -> ()  [unwired: 1 in, 5 out]
                n147 = Select(t=T4."Enabled" ("Disabled"), s="OwningLibrary_chkBox", f=T4."Disabled and Grayed Out") -> (s? t:f=w533:T4)
                n148 = property on="Name of Owning Library" class="Str"(error in=w528, "DisabledEnum"=w533) -> (error out=w531:errorcluster)  [unwired: 1 in, 1 out]
                n149 = property on="Path to Owning Library" class="Str"(error in=w528, "DisabledEnum"=w533) -> (error out=w530:errorcluster)  [unwired: 1 in, 1 out]
                n150 = Bundle By Name(cluster=w522, "IsOwningLibraryON?"="OwningLibrary_chkBox") -> (w519:T1)
                n151 = Build Array(w531, w530) -> (w518:errorcluster[])
                n152 = Merge Errors(w518) -> (w526:errorcluster)
                n153 = Enqueue Element(queue=w527, element=UserDialogStates."Update" ("UserDialogSteps"), error in (no error)=w526) -> (queue out=w524:refnum<queue>, error out=w523:errorcluster)  [unwired: 1 in, 1 out]
              }
              event "Details_chkBox": Value Change {
                n154 = event-data() -> ()  [unwired: 1 in, 5 out]
                n155 = Select(t=T4."Enabled" ("Disabled"), s="Details_chkBox", f=T4."Disabled and Grayed Out") -> (s? t:f=w549:T4)
                n156 = Bundle By Name(cluster=w539, "IsDetailsON?"="Details_chkBox") -> (w536:T1)
                n157 = property on="Details" class="Str"(error in=w544, "DisabledEnum"=w549) -> (error out=w543:errorcluster)  [unwired: 1 in, 1 out]
                n158 = Enqueue Element(queue=w545, element=UserDialogStates."Update" ("UserDialogSteps"), error in (no error)=w543) -> (queue out=w541:refnum<queue>, error out=w540:errorcluster)  [unwired: 1 in, 1 out]
              }
              event "Examples_chkBox": Value Change {
                n159 = event-data() -> ()  [unwired: 1 in, 5 out]
                n160 = Select(t=T4."Enabled" ("Disabled"), s="Examples_chkBox", f=T4."Disabled and Grayed Out") -> (s? t:f=w563:T4)
                n161 = property on="Example VI name" class="Str"(error in=w559, "DisabledEnum"=w563) -> (error out=w567:errorcluster)  [unwired: 1 in, 1 out]
                n162 = property on="Example VI Path" class="Path"(error in=w559, "DisabledEnum"=w563) -> (error out=w566:errorcluster)  [unwired: 1 in, 1 out]
                n163 = property on="Image Path for Example" class="Str"(error in=w559, "DisabledEnum"=w563) -> (error out=w562:errorcluster)  [unwired: 1 in, 1 out]
                n164 = Bundle By Name(cluster=w555, "IsExamplesON?"="Examples_chkBox") -> (w552:T1)
                n165 = Build Array(w567, w566, w562) -> (w551:errorcluster[])
                n166 = Merge Errors(w551) -> (w560:errorcluster)
                n167 = Enqueue Element(queue=w561, element=UserDialogStates."Update" ("UserDialogSteps"), error in (no error)=w560) -> (queue out=w557:refnum<queue>, error out=w556:errorcluster)  [unwired: 1 in, 1 out]
              }
              event "Help Button": Value Change {
                n168 = event-data() -> ()  [unwired: 1 in, 5 out]
                n169 = call "Read me and Help.vi"("path"=path "viGods.com/HELPer/advanced.html", "error in"=w578) -> ("error out"=w576:errorcluster)  [unwired: 13 in]
                n170 = Enqueue Element(queue=w575, element=UserDialogStates."Update" ("UserDialogSteps"), error in (no error)=w576) -> (queue out=w573:refnum<queue>, error out=w572:errorcluster)  [unwired: 1 in, 1 out]
              }
              event "www.labicom.net": Value Change {
                n171 = event-data() -> ()  [unwired: 1 in, 5 out]
                n172 = call-poly <vilib>:"Open URL in Default Browser.vi"("error in (no error)"=w591, "URL"="https://labicom.net/labdeveloper/helper/") -> ("error out"=w587:errorcluster)  [unwired: 4 in, 1 out]
                n173 = Enqueue Element(queue=w586, element=UserDialogStates."Update" ("UserDialogSteps"), error in (no error)=w587) -> (queue out=w584:refnum<queue>, error out=w583:errorcluster)  [unwired: 1 in, 1 out]
              }
              event "Cancel Button": Value Change {
                n174 = event-data() -> ()  [unwired: 1 in, 5 out]
                n175 = Not(x="Cancel Button") -> (.not. x?=w599:bool)
                n176 = local write "Cancel Button"(w599) -> ()
                n177 = Enqueue Element(queue=w597, element=UserDialogStates."Shutdown" ("UserDialogSteps"), error in (no error)=w598) -> (queue out=w596:refnum<queue>, error out=w595:errorcluster)  [unwired: 1 in, 1 out]
                "Cancelled by User?" <- TRUE ("Cancelled by User?")
              }
            }
          }
          frame "Update" {
            n178 = Enqueue Element(queue=w613, element=UserDialogStates."Choose parameters", error in (no error)=w614) -> (queue out=w611:refnum<queue>, error out=w610:errorcluster)  [unwired: 1 in, 1 out]
          }
          frame "Shutdown" {
            n179 = case shown="False" w622 {
              tunnel: [w656 TRUE] -> w633
              tunnel: w616 -> [w655 w757]
              tunnel: w632 -> [w654 w760]
              tunnel: w631 -> [w653 w761]
              tunnel: [w652 w761] -> w630
              tunnel: [w651 w756] -> w629
              tunnel: w628 -> [w650 w759]
              tunnel: [w648 w753] -> w627
              tunnel: [w647 w760] -> w626
              tunnel: [w646 w759] -> w625
              tunnel: w624 -> [w643 w762]
              tunnel: [w644 w762] -> w623
              tunnel: w621 -> [_ _]
              tunnel: w618 -> [w640 _]
              tunnel: w620 -> [w638 w758]
              tunnel: w618 -> [w637 _]
              tunnel: w619 -> [w636 _]
              tunnel: [w635 TRUE ("IsScrollableDetails?")] -> w617
              tunnel: w615 -> [w634 w754]
              frame False {
                # "> VI Name >"
                n180 = Concatenate Strings(w640, ".html" ("string")) -> (w639:string)
                n181 = Not(x=w643) -> (.not. x?=w642:bool)
                n182 = call "_UserDialog Choose Filename.vi"("VI Default Path"=w650, "Default file name"=w639, "Not In <help> directory? (Yes: T)"=w642) -> ("HTML File Path"=w649:path, "Cancelled by User?"=w645:bool)  [unwired: 8 in, 3 out]
                n183 = case shown="False" w645 {
                  tunnel: [TRUE FALSE] -> w656
                  tunnel: w655 -> [w669 w742]
                  tunnel: w654 -> [w662 w748]
                  tunnel: w653 -> [w692 w749]
                  tunnel: [w690 w749] -> w652
                  tunnel: [w688 w741] -> w651
                  tunnel: w649 -> [w671 w747]
                  tunnel: [w659 w744] -> w648
                  tunnel: [w662 w748] -> w647
                  tunnel: [w671 w747] -> w646
                  tunnel: w643 -> [w674 w750]
                  tunnel: [w674 w750] -> w644
                  tunnel: w638 -> [w673 _]
                  tunnel: w637 -> [w667 _]
                  tunnel: w636 -> [w666 _]
                  tunnel: [w658 TRUE ("IsScrollableDetails?")] -> w635
                  tunnel: w634 -> [w660 w745]
                  frame False {
                    # "> HTML file path >"
                    # "> Documented VI path >"
                    # "> HTML file path >"
                    # "Clear error 7 'File not found'"
                    n184 = local read "IsDetailedHelpLink?"() -> (w705:bool)
                    n185 = local read "Start path location"() -> (w663:T2)
                    n186 = case shown="True" w705 {
                      tunnel: [path "" w714] -> w700
                      tunnel: w671 -> [_ w713]
                      tunnel: [w707 w712] -> w699
                      tunnel: w669 -> [w707 w710]
                      tunnel: w663 -> [_ w711]
                      tunnel: w662 -> [_ w709]
                      frame False {
                      }
                      frame True {
                        # "> VI path >"
                        # "> HTML path >"
                        # "User chose to have 'Detailed Help' link"
                        n187 = case shown="\"VI folder\", Default" w711 {
                          tunnel: [w718 w730] -> w714
                          tunnel: w713 -> [w715 w729]
                          tunnel: [w717 w726] -> w712
                          tunnel: w710 -> [w724 w725]
                          tunnel: w709 -> [w716 _]
                          frame "VI folder", Default {
                            # "Replace absolute path to HTML \nhelp file with relative path \n(relative to documented VI)"
                            n188 = call <vilib>:"Compare Two Paths.vi"("error in (no error)"=w724, "Path 2"=w715, "Path 1"=w716) -> ("error out"=w720:errorcluster, "Relative Path from 1 to 2"=w721:path)  [unwired: 5 in, 2 out]
                            n189 = Path To String(path=w721) -> (string=w723:string)
                            n190 = Search and Replace String(input string=w723, search string="..\\", error in=w720) -> (result string=w719:string, error out=w717:errorcluster)  [unwired: 5 in, 2 out]
                            n191 = String To Path(string=w719) -> (path=w718:path)
                          }
                          frame "Help folder" {
                            # "Replace absolute path to LabVIEW \nhelp folder with symbolic path \n'<helpdir>:\\'"
                            n192 = Open Application Reference(8:w725) -> (0:w739:errorcluster, 3:w740:refnum<vi>)  [unwired: 3 in]
                            n193 = property class="App"(reference=w740, error in=w739) -> (reference out=w738:refnum<vi>, error out=w737:errorcluster, "App.Dir"=w736:path)
                            n194 = Close Reference(reference=w738, error in (no error)=w737) -> (error out=w727:errorcluster)
                            n195 = Build Path(base path=w736, name or relative path="help") -> (appended path=w728:path)
                            n196 = Path To String(path=w728) -> (string=w732:string)
                            n197 = Path To String(path=w729) -> (string=w731:string)
                            n198 = Search and Replace String(input string=w731, search string=w732, replace string="<helpdir>:\\" ("replace string (\"\")"), error in=w727) -> (result string=w734:string, error out=w726:errorcluster)  [unwired: 4 in, 2 out]
                            n199 = String To Path(string=w734) -> (path=w730:path)
                          }
                        }
                      }
                    }
                    n200 = Unbundle By Name(w692) -> ("_owning_library_html_"=w698:string, "_example_screenshot_"=w677:string)
                    n201 = call "_Create HTML file and folders.vi"("Menu Launch:App"=w666, "HTML File Path"=w671, "Menu Launch:VI"=w667, "error in (no error)"=w669) -> ("HTML FIle Path out"=w670:path, "error out"=w668:errorcluster)  [unwired: 10 in]
                    n202 = String To Path(string=w677) -> (path=w676:path)
                    n203 = String To Path(string=w698) -> (path=w693:path)
                    n204 = Strip Path(path=w670) -> (stripped path=w686:path, name=w684:string)
                    n205 = Concatenate Strings(w684, "_Images" ("name or relative path")) -> (w683:string)
                    n206 = call <vilib>:"Compare Two Paths.vi"("error in (no error)"=w668, "Path 2"=w693, "Path 1"=w671) -> ("error out"=w697:errorcluster, "Relative Path from 1 to 2"=w696:path)  [unwired: 5 in, 2 out]
                    n207 = Path To String(path=w696) -> (string=w695:string)
                    n208 = Build Path(base path=w686, name or relative path=w683) -> (appended path=w687:path)
                    n209 = Strip Path(path=w676) -> (name=w681:string)  [unwired: 1 out]
                    n210 = Strip Path(path=w687) -> (name=w680:string)  [unwired: 1 out]
                    n211 = Search and Replace String(input string=w695, search string="..\\", error in=w697) -> (result string=w691:string, error out=w672:errorcluster)  [unwired: 5 in, 2 out]
                    n212 = Build Path(base path=w687, name or relative path=w681) -> (appended path=w678:path)
                    n213 = Copy(8:w672, 9:TRUE ("overwrite (F)"), 10:w678, 11:w676) -> (0:w665:errorcluster)  [unwired: 1 in, 2 out]
                    n214 = property class="VI"(reference=w673, error in=w699, "Help.Path"=w700) -> (reference out=w704:refnum<vi>, error out=w702:errorcluster)
                    n215 = Concatenate Strings(w680, "/" ("string"), w681) -> (w675:string)
                    n216 = Bundle By Name(cluster=w692, "_owning_library_html_"=w691, "_example_screenshot_"=w675) -> (w690:T1)
                    n217 = invoke class="VI" method="Save.Instrument"(reference=w704, error in=w702, "Path to saved file"=w662) -> (reference out=w703:refnum<vi>, error out=w701:errorcluster)  [unwired: 3 in, 4 out]
                    n218 = local read "IsScrollableDetails?"() -> (w658:bool)
                    n219 = call <vilib>:"Clear Errors.vi"("error in (no error)"=w665) -> ("error out"=w664:errorcluster)  [unwired: 6 in]
                    n220 = Enqueue Element(queue=w660, element=UserDialogStates."Shutdown" ("UserDialogSteps")) -> (queue out=w659:refnum<queue>)  [unwired: 2 in, 2 out]
                    n221 = Close Reference(reference=w703, error in (no error)=w701) -> (error out=w689:errorcluster)
                    n222 = Build Array(w689, w664) -> (w657:errorcluster[])
                    n223 = Merge Errors(w657) -> (w688:errorcluster)
                  }
                  frame True {
                    # "Cancelled by user in the file path dialog"
                    n224 = Enqueue Element(queue=w745, element=UserDialogStates."Choose parameters" ("UserDialogSteps"), error in (no error)=w742) -> (queue out=w744:refnum<queue>, error out=w741:errorcluster)  [unwired: 1 in, 1 out]
                  }
                }
              }
              frame True {
                # "Cancelled by user permanently"
                n225 = Close Reference(reference=w758, error in (no error)=w757) -> (error out=w756:errorcluster)
                n226 = Enqueue Element(queue=w754, element=UserDialogStates."Shutdown" ("UserDialogSteps")) -> (queue out=w753:refnum<queue>)  [unwired: 2 in, 2 out]
              }
            }
          }
        }
      }
      "HTML File Path" <- w32
      n227 = local read "Cancelled by User?"() -> (w36:bool)
      n228 = case shown="True" w17 {
        tunnel: ["<HTML>\n<HEAD>\n<TITLE>_vi_name_</TITLE>\n<link rel=\"stylesheet\" type=\"text/css\" href=\"Resources/help.css\">\n<META NAME=\"Author\" CONTENT=\"\">\n<META NAME=\"GENERATOR\" CONTENT=\"HELPer - VI Documentation Toolkit from www.vigods.com\">\n</HEAD>\n<BODY>\n<A NAME=\"_vi_name_\"></A><H1>_vi_name_</H1>\n\n<!--Owning Palette-->\n\n<p class=\"Body\"><strong>Owning Palette:</strong> <a href=\"_owning_library_html_\">_name_of_owning_library_</a></p>\n\n<!--Package-->\n\n<p class=\"Body\"><strong>Requires:</strong> _Packages_</p>\n\n<!--Platform-->\n\n<p class=\"Body\"><strong>Platform(s):</strong> _Platforms_</p>\n\n<!-- VI/Function Description -->\n\n<p class=\"Body\">_vi_description_text_</p>\n\n<!-- Supplemental VI/Function Information -->\n\n\n\n<!-- Link to Additional VI/Function Information and Examples  -->\n\n<p class=\"Body\"><a href=\"#details\">Details</a>&nbsp;&nbsp;<a href=\"#examples\">Example</a></p>\n\n\n<!-- Graphic Reference -->\n\n<p class=\"Anchor\"><IMG SRC=\"_images_folder_path_/_vi_connector_pane_c.png\" ALT=\"_vi_name_\" border=\"1\" style=\"margin: 2px; padding: 5px\"></p>\n<hr>\n\n<div id=\"styleDivScrolling\">\n\n<!-- Table of VI/Function Parameters -->\n\n_vi_controls_and_indicators_descriptions_\n\n<!-- Table of VI Descriptions -->\n<table class=\"Bordered\">\n<tr>\n\t<th class=\"Bordered Left-Align\">Object</th>\n\t<th class=\"Bordered Left-Align\">Description</th>\n</tr>\n_vis_descriptions_table_\n</table>\n\n<!-- Additional VI/Function Information -->\n\n<h2><a name=\"details\">Details</a></h2>\n<p class=\"Body\">_details_text_</p>\n\n<!-- Example Information -->\n\n<h2><a name=\"examples\">Example</a></h2>\n<p class=\"Anchor\"><IMG SRC=\"_example_screenshot_\"></p>\n<p class=\"Body\">Refer to the <strong>_example_vi_</strong> VI in the <span class=\"Monospace\">_path_to_example_file_</span> for an example of using the <strong>_vi_name_</strong>.</p>\n\n</div>\n</BODY>\n</HTML>" w41] -> w18
        frame False {
          # "Not scrollable"
        }
        frame True {
          w41 = "<HTML>\n<HEAD>\n<TITLE>_vi_name_</TITLE>\n<link rel=\"stylesheet\" type=\"text/css\" href=\"Resources/help.css\">\n<META NAME=\"Author\" CONTENT=\"\">\n<META NAME=\"GENERATOR\" CONTENT=\"VI HELPer Documentation Toolkit from https://labicom.net/labdeveloper/helper/\">\n</HEAD>\n<BODY>\n<div id=\"notScrollable\">\n<A NAME=\"_vi_name_\"></A><H1>_vi_name_</H1>\n\n<!--Owning Palette-->\n\n<p class=\"Body\"><strong>Owning Palette:</strong> <a href=\"_owning_library_html_\">_name_of_owning_library_</a></p>\n\n<!--Package-->\n\n<p class=\"Body\"><strong>Requires:</strong> _Packages_</p>\n\n<!--Platform-->\n\n<p class=\"Body\"><strong>Platform(s):</strong> _Platforms_</p>\n\n<!-- VI/Function Description -->\n\n<p class=\"Body\">_vi_description_text_</p>\n\n<!-- Supplemental VI/Function Information -->\n\n\n\n<!-- Link to Additional VI/Function Information and Examples  -->\n\n<p class=\"Body\"><a href=\"#details\">Details</a>&nbsp;&nbsp;<a href=\"#examples\">Example</a></p>\n\n\n<!-- Graphic Reference -->\n\n<p class=\"Anchor\"><IMG SRC=\"_images_folder_path_/_vi_connector_pane_c.png\" ALT=\"_vi_name_\" border=\"1\" style=\"margin: 2px; padding: 5px\"></p>\n<hr>\n</div>\n\n<div id=\"styleDivScrolling\" style=\"overflow: auto;>\n\n<!-- Table of VI/Function Parameters -->\n\n_vi_controls_and_indicators_descriptions_\n\n<!-- Table of VI Descriptions -->\n<table class=\"Bordered\">\n<tr>\n\t<th class=\"Bordered Left-Align\">Object</th>\n\t<th class=\"Bordered Left-Align\">Description</th>\n</tr>\n_vis_descriptions_table_\n</table>\n\n<!-- Additional VI/Function Information -->\n\n<h2><a name=\"details\">Details</a></h2>\n<p class=\"Body\">_details_text_</p>\n\n<!-- Example Information -->\n\n<h2><a name=\"examples\">Example</a></h2>\n<p class=\"Anchor\"><IMG SRC=\"_example_screenshot_\"></p>\n<p class=\"Body\">Refer to the <strong>_example_vi_</strong> VI in the <span class=\"Monospace\">_path_to_example_file_</span> for an example of using the <strong>_vi_name_</strong>.</p>\n\n</div>\n<script>\n\tvar notScrollableHeight = document.getElementById(\"notScrollable\").offsetHeight;\n\tvar browserWindowHeight = window.innerHeight;\n\tstyleDivScrolling.style.height = browserWindowHeight - notScrollableHeight - 18;\n</script>\n</BODY>\n</HTML>"  # <HTML> <HEAD> <TITLE>_vi_name_</TITLE> <link rel="stylesheet" type="text/css" href="Resources/help.css"> <META NAME="Author" CONTENT=""> <META NAME="GENERATOR" CONTENT="VI HELPer Documentation Toolkit from https://labicom.net/labdeveloper/helper/"> </HEAD> <BODY> <div id="notScrollable"> <A NAME="_vi_name_"></A><H1>_vi_name_</H1>  <!--Owning Palette-->  <p class="Body"><strong>Owning Palette:</strong> <a href="_owning_library_html_">_name_of_owning_library_</a></p>  <!--Package-->  <p class="Body"><strong>Requires:</strong> _Packages_</p>  <!--Platform-->  <p class="Body"><strong>Platform(s):</strong> _Platforms_</p>  <!-- VI/Function Description -->  <p class="Body">_vi_description_text_</p>  <!-- Supplemental VI/Function Information -->    <!-- Link to Additional VI/Function Information and Examples  -->  <p class="Body"><a href="#details">Details</a>&nbsp;&nbsp;<a href="#examples">Example</a></p>   <!-- Graphic Reference -->  <p class="Anchor"><IMG SRC="_images_folder_path_/_vi_connector_pane_c.png" ALT="_vi_name_" border="1" style="margin: 2px; padding: 5px"></p> <hr> </div>  <div id="styleDivScrolling" style="overflow: auto;>  <!-- Table of VI/Function Parameters -->  _vi_controls_and_indicators_descriptions_  <!-- Table of VI Descriptions --> <table class="Bordered"> <tr> 	<th class="Bordered Left-Align">Object</th> 	<th class="Bordered Left-Align">Description</th> </tr> _vis_descriptions_table_ </table>  <!-- Additional VI/Function Information -->  <h2><a name="details">Details</a></h2> <p class="Body">_details_text_</p>  <!-- Example Information -->  <h2><a name="examples">Example</a></h2> <p class="Anchor"><IMG SRC="_example_screenshot_"></p> <p class="Body">Refer to the <strong>_example_vi_</strong> VI in the <span class="Monospace">_path_to_example_file_</span> for an example of using the <strong>_vi_name_</strong>.</p>  </div> <script> 	var notScrollableHeight = document.getElementById("notScrollable").offsetHeight; 	var browserWindowHeight = window.innerHeight; 	styleDivScrolling.style.height = browserWindowHeight - notScrollableHeight - 18; </script> </BODY> </HTML>
          # "Scrollable"
        }
      }
      n229 = case shown="False" w36 {
        tunnel: w33 -> [w52 w70]
        tunnel: w35 -> [w54 _]
        tunnel: [w43 w70] -> w34
        tunnel: w18 -> [w66 _]
        tunnel: w32 -> [w53 _]
        tunnel: w24 -> [_ _]
        frame False {
          # "Extract control/indicator descriptions\nfrom 'VI Print'ed LabVIEW method"
          # "Add line feeds (LFs) after each control/indicator\ndescription for better layout and structure of html\nsource file"
          n230 = Read from Text File(file (use dialog)=w53, count=-1, error in=w52) -> (refnum out=w60:refnum<file>, text=w64:string, error out=w59:errorcluster)  [unwired: 1 in, 1 out]
          n231 = Match Pattern(string=w64, regular expression="\"></P>" ("search string")) -> (after substring=w62:string)  [unwired: 1 in, 3 out]
          n232 = Close File(refnum=w60, error in=w59) -> (path=w55:path, error out=w56:errorcluster)
          n233 = Match Pattern(string=w62, regular expression="</BODY>") -> (before substring=w51:string)  [unwired: 1 in, 3 out]
          n234 = Concatenate Strings("</TD>" ("replace string (\"\")"), "\r") -> (w46:string)
          n235 = Search and Replace String(replace all?=TRUE ("replace all? (F)"), input string=w51, search string="</TD>", replace string=w46) -> (result string=w45:string)  [unwired: 4 in, 3 out]
          n236 = Bundle By Name(cluster=w54, "_vi_controls_and_indicators_descriptions_"=w45) -> (w57:T1)
          n237 = Write to Text File(file (use dialog)=w55, text=w66, error in=w56) -> (refnum out=w68:refnum<file>, error out=w69:errorcluster)  [unwired: 1 in, 1 out]
          n238 = Close File(refnum=w68, error in=w69) -> (path=w67:path, error out=w65:errorcluster)
          n239 = call "_Postprocess HTML file.vi"("HTML File Path"=w67, "VI Info"=w57, "error in"=w65) -> ("HTML File Path out"=w42:path, "error out"=w44:errorcluster)  [unwired: 11 in]
          n240 = call-poly <vilib>:"Open URL in Default Browser.vi"("error in (no error)"=w44, "path"=w42) -> ("error out"=w43:errorcluster)  [unwired: 4 in, 1 out]
        }
        frame True {
          # "Cancelled by User"
          n241 = local write "Cancelled by User?"(FALSE ("Cancelled by User?")) -> ()
        }
      }
    }
    frame Error {
      n242 = Close Reference(reference=w765, error in (no error)=w766) -> (error out=w764:errorcluster)
    }
  }
  n243 = call <vilib>:"Clear Errors.vi"("error in (no error)"=w2) -> ("error out"=w1:errorcluster)  [unwired: 6 in]
  n244 = control-ref of="This VI"() -> (w6:refnum<vi>)
  n245 = invoke class="VI" method="FP.Close"(reference=w6, error in=w1) -> (reference out=w4:refnum<vi>, error out=w5:errorcluster)  [unwired: 1 in, 1 out]
  n246 = Close Reference(reference=w4, error in (no error)=w5) -> (error out=→"error out":errorcluster)
